vi "Update(Camera).vi"(8 "error in (no error)":errorcluster, 10 "Camera_Settings":T2 {"WhiteB." min=2000 max=7500 step=1; "Gain" max=255 step=5; "Exposure" min=0 max=9 step=5; "Focus" step=5}, 11 "Session in":T1) -> (0 "error out":errorcluster, 3 "Session out":T1)   [LabVIEW 2024]
uses:
  Controls/Camera_Settings.ctl
  <vilib>/userDefined/High Color/IMAQdx.ctl
  1c965d0a-2fbf-4a15-954e-c94853878a6e.vi
  <resource>/objmgr/imaqdx.rc
  <vilib>/vision/driver/NI_Vision_Acquisition_Software.lvlib
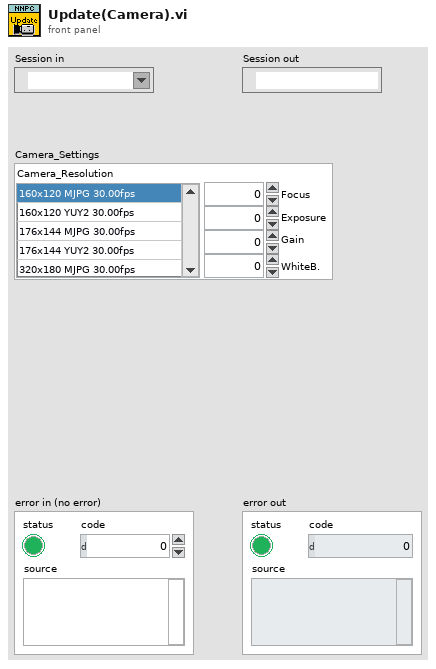
[diagram p1: front panel]
types:
  T1 = typedef "IMAQdx.ctl" = refnum<k21>
  T2 = typedef "Camera_Settings.ctl" = cluster{"Camera_Resolution":i32, "Focus":u8, "Exposure":i32, "Gain":u32, "WhiteB.":i32}
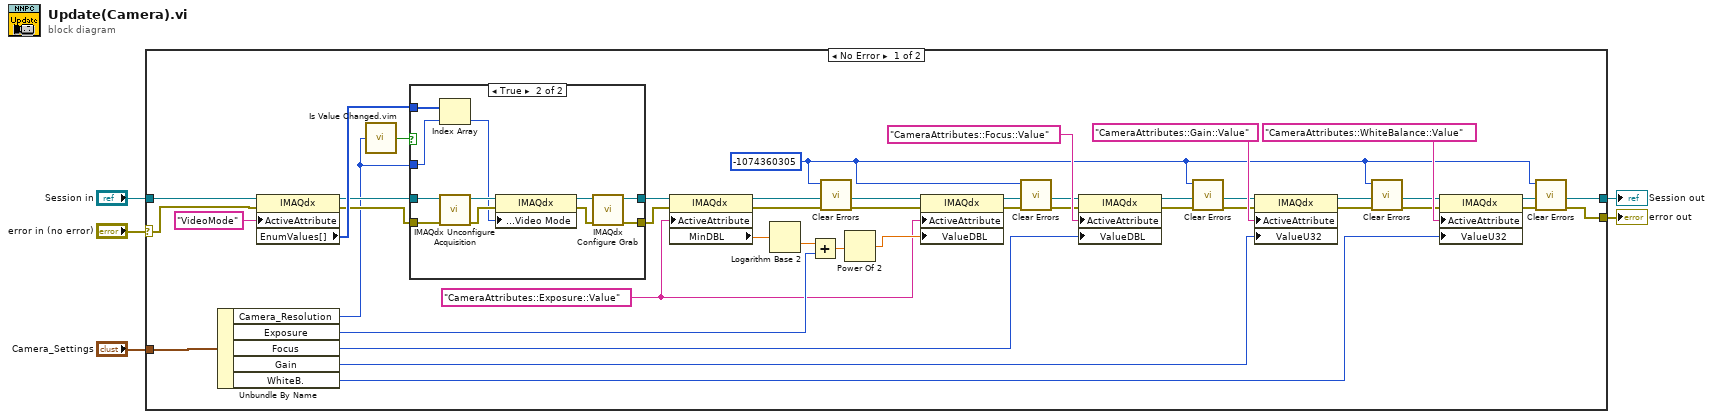
[diagram p0: block diagram]
diagram:
  n1 = case shown="No Error" "error in (no error)" {
    selector: "error in (no error)" -> [w39 w59]
    tunnel: "Session in" -> [w40 w58]
    tunnel: "Camera_Settings" -> [w35 _]
    tunnel: [w13 w58] -> w2
    tunnel: [w11 w59] -> w1
    frame No Error {
      w6 = -1074360305 ("specific error code to clear (0: all)")
      w27 = "CameraAttributes::Exposure::Value" ("ActiveAttribute")
      n2 = Unbundle By Name(w35) -> ("Camera_Resolution"=w34:i32, "Exposure"=w44:i32, "Focus"=w24:u8, "Gain"=w21:u32, "WhiteB."=w18:i32)
      n3 = property class="IMAQdx"(reference=w40, error in=w39, "ActiveAttribute"="VideoMode") -> (reference out=w37:T1, error out=w36:errorcluster, "EnumValues[]"=w38:u32[])
      n4 = call "Is Value Changed.vim"("value"=w34) -> ("changed or first call?"=w41:bool)
      n5 = case shown="True" w41 {
        tunnel: [w46 w53] -> w32
        tunnel: [w45 w54] -> w31
        tunnel: w38 -> [_ w57]
        tunnel: w34 -> [_ w56]
        tunnel: w36 -> [w45 w48]
        tunnel: w37 -> [w46 w47]
        frame False {
        }
        frame True {
          n6 = Index Array(array=w57, index=w56) -> (element=w49:u32)
          n7 = call <vilib>:"IMAQdx Unconfigure Acquisition.vi"("error in"=w48, "Session In"=w47) -> ("error out"=w50:errorcluster, "Session Out"=w55:T1)  [unwired: 8 out]
          n8 = property class="IMAQdx"(reference=w55, error in=w50, "Acquisition Attributes:Video Mode"=w49) -> (reference out=w52:T1, error out=w51:errorcluster)
          n9 = call <vilib>:"IMAQdx Configure Grab.vi"("error in"=w51, "Session In"=w52) -> ("error out"=w54:errorcluster, "Session Out"=w53:T1)  [unwired: 2 in, 6 out]
        }
      }
      n10 = property class="IMAQdx"(reference=w32, error in=w31, "ActiveAttribute"=w27) -> (reference out=w17:T1, error out=w29:errorcluster, "MinDBL"=w30:dbl)
      n11 = Logarithm Base 2(1:w30) -> (0:w42:dbl)
      n12 = Add(x=w42, y=w44) -> (x+y=w43:dbl)
      n13 = call <vilib>:"Clear Errors.vi"("error in (no error)"=w29, "specific error code to clear (0: all)"=w6) -> ("error out"=w7:errorcluster)  [unwired: 4 in, 1 out]
      n14 = Power Of 2(x=w43) -> (2^x=w28:dbl)
      n15 = property class="IMAQdx"(reference=w17, error in=w7, "ActiveAttribute"=w27, "ValueDBL"=w28) -> (reference out=w16:T1, error out=w25:errorcluster)
      n16 = call <vilib>:"Clear Errors.vi"("error in (no error)"=w25, "specific error code to clear (0: all)"=w6) -> ("error out"=w8:errorcluster)  [unwired: 4 in, 1 out]
      n17 = property class="IMAQdx"(reference=w16, error in=w8, "ActiveAttribute"="CameraAttributes::Focus::Value", "ValueDBL"=w24) -> (reference out=w15:T1, error out=w22:errorcluster)
      n18 = call <vilib>:"Clear Errors.vi"("error in (no error)"=w22, "specific error code to clear (0: all)"=w6) -> ("error out"=w9:errorcluster)  [unwired: 4 in, 1 out]
      n19 = property class="IMAQdx"(reference=w15, error in=w9, "ActiveAttribute"="CameraAttributes::Gain::Value", "ValueU32"=w21) -> (reference out=w14:T1, error out=w19:errorcluster)
      n20 = call <vilib>:"Clear Errors.vi"("error in (no error)"=w19, "specific error code to clear (0: all)"=w6) -> ("error out"=w10:errorcluster)  [unwired: 4 in, 1 out]
      n21 = property class="IMAQdx"(reference=w14, error in=w10, "ActiveAttribute"="CameraAttributes::WhiteBalance::Value", "ValueU32"=w18) -> (reference out=w13:T1, error out=w12:errorcluster)
      n22 = call <vilib>:"Clear Errors.vi"("error in (no error)"=w12, "specific error code to clear (0: all)"=w6) -> ("error out"=w11:errorcluster)  [unwired: 4 in, 1 out]
    }
    frame Error {
    }
  }
  "Session out" <- w2
  "error out" <- w1
